vi "ConfigureSystemDefinitionFile.vi"(8 "error in (no error)":errorcluster, 9 "Target Rate":dbl, 10 "Destination System Definition File in":path, 11 "Source System Definition File in":path) -> (0 "error out":errorcluster)   [LabVIEW 2027, in "VeriStandTestUtilities.lvlib"]
uses:
  VeriStandTestUtilities.lvlib
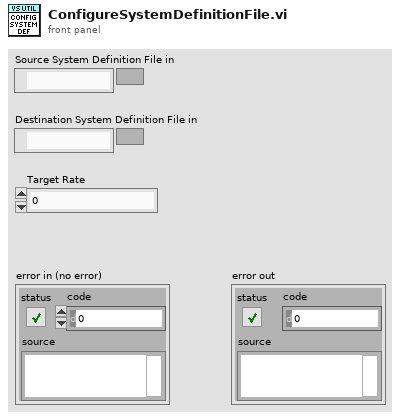
[diagram p1: front panel]
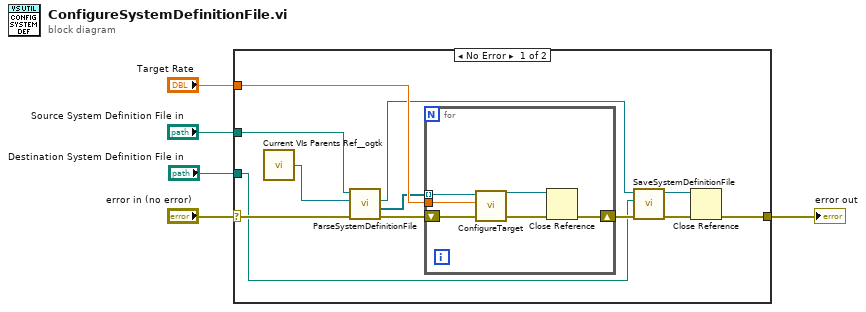
[diagram p0: block diagram]
diagram:
  n1 = case shown="No Error" "error in (no error)" {
    selector: "error in (no error)" -> [w17 w24]
    tunnel: [w10 w24] -> w4
    tunnel: "Source System Definition File in" -> [w15 _]
    tunnel: "Target Rate" -> [w12 _]
    tunnel: "Destination System Definition File in" -> [w6 _]
    frame No Error {
      n2 = call <userlib>:"Current VIs Parents Ref__ogtk.vi"() -> ("Calling VI's Reference"=w16:refnum<vi>)  [unwired: 2 in]
      n3 = call "ParseSystemDefinitionFile.vi"("error in (no error)"=w17, "VI in"=w16, "System Definiton File in"=w15) -> ("error out"=w14:errorcluster, "Target List out"=w11:refnum<k39>[], "NationalInstruments.VeriStand.SystemDefinitionAPI.SystemDefinition"=w8:refnum<k39>)  [unwired: 5 in, 1 out]
      n4 = for {
        shift-right: [w23] -> w13
        shift-left: w14 -> [w21]
        tunnel: w12 -> [w19]
        tunnel: w11 -> [w18] mode=indexing
        n5 = call "ConfigureTarget.vi"("error in (no error)"=w21, "TargetRate"=w19, "NationalInstruments.VeriStand.SystemDefinitionAPI.Target"=w18) -> ("error out"=w20:errorcluster, "NationalInstruments.VeriStand.SystemDefinitionAPI.Target"=w22:refnum<k39>)  [unwired: 7 in]
        n6 = Close Reference(reference=w22, error in (no error)=w20) -> (error out=w23:errorcluster)
      }
      n7 = call "SaveSystemDefinitionFile.vi"("error in (no error)"=w13, "System Definition File in"=w6, "NationalInstruments.VeriStand.SystemDefinitionAPI.SystemDefinition"=w8) -> ("error out"=w9:errorcluster, "NationalInstruments.VeriStand.SystemDefinitionAPI.SystemDefinition"=w7:refnum<k39>)  [unwired: 7 in]
      n8 = Close Reference(reference=w7, error in (no error)=w9) -> (error out=w10:errorcluster)
    }
    frame Error {
    }
  }
  "error out" <- w4
